vi "SelectStageTrajectory2.vi"(6 "Stage Position Limit":i32=360, 9 "Stage Speed":dbl=45.0 format="%#_13g", 10 "New Stage Position":i32, 11 "Stage Position":dbl) -> ()   [LabVIEW 2013]
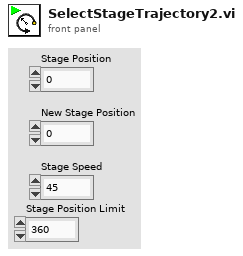
[diagram p1: front panel]
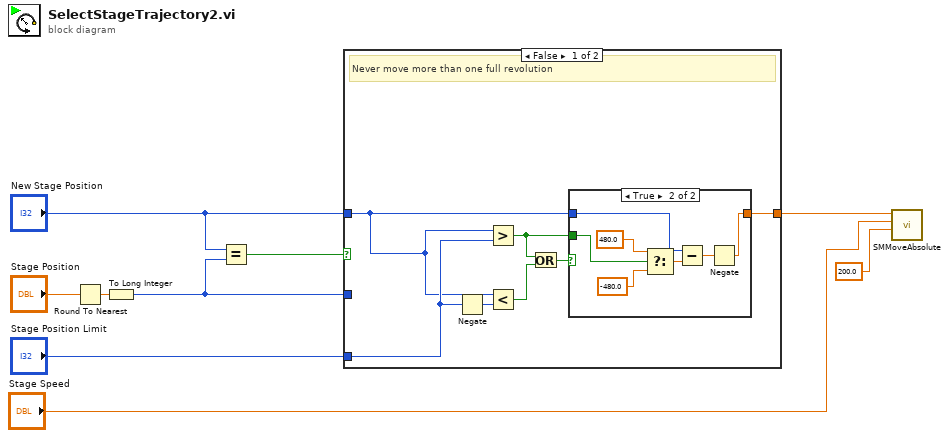
[diagram p0: block diagram]
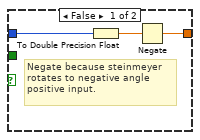
[diagram p2: hidden frame]
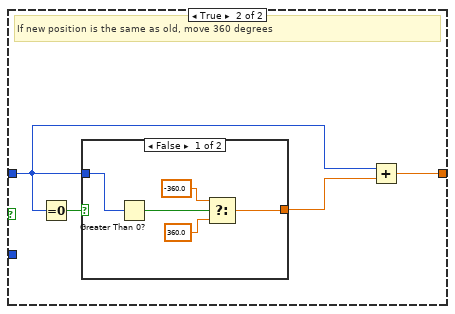
[diagram p3: hidden frame]
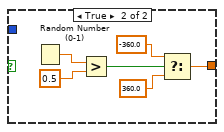
[diagram p4: hidden frame]
diagram:
  n1 = Round To Nearest(number="Stage Position") -> (nearest integer value=w7:dbl)
  n2 = To Long Integer(number=w7) -> (32bit integer=w4:i32)
  n3 = Equal?(x="New Stage Position", y=w4) -> (x = y?=w6:bool)
  n4 = case shown="False" w6 {
    tunnel: "New Stage Position" -> [w10 w28]
    tunnel: [w13 w27] -> w3
    tunnel: w4 -> [_ _]
    tunnel: "Stage Position Limit" -> [w12 _]
    frame False {
      # "Never move more than one full revolution"
      n5 = Negate(x=w12) -> (-x=w11:i32)
      n6 = Greater?(x=w10, y=w12) -> (0:w14:bool)
      n7 = Less?(x=w10, y=w11) -> (x < y?=w15:bool)
      n8 = Or(x=w14, y=w15) -> (x .or. y?=w16:bool)
      n9 = case shown="True" w16 {
        tunnel: w14 -> [_ w24]
        tunnel: w10 -> [w19 w23]
        tunnel: [w17 w20] -> w13
        frame False {
          # "Negate because steinmeyer \nrotates to negative angle \npositive input."
          n10 = To Double Precision Float(number=w19) -> (double precision float=w18:dbl)
          n11 = Negate(x=w18) -> (-x=w17:dbl)
        }
        frame True {
          n12 = Select(t=480.0, s=w24, f=-480.0) -> (s? t:f=w22:dbl)
          n13 = Subtract(x=w23, y=w22) -> (x-y=w21:dbl)
          n14 = Negate(x=w21) -> (-x=w20:dbl)
        }
      }
    }
    frame True {
      # "If new position is the same as old, move 360 degrees"
      n15 = Equal To 0?(x=w28) -> (x = 0?=w30:bool)
      n16 = case shown="False" w30 {
        tunnel: w28 -> [w35 _]
        tunnel: [w31 w36] -> w29
        frame False {
          n17 = Greater Than 0?(x=w35) -> (x > 0?=w32:bool)
          n18 = Select(t=-360.0, s=w32, f=360.0) -> (s? t:f=w31:dbl)
        }
        frame True {
          n19 = Random Number (0-1)() -> (number: 0 to 1=w41:dbl)
          n20 = Greater?(x=w41, y=0.5) -> (0:w37:bool)
          n21 = Select(t=-360.0, s=w37, f=360.0) -> (s? t:f=w36:dbl)
        }
      }
      n22 = Add(x=w28, y=w29) -> (x+y=w27:dbl)
    }
  }
  n23 = call "SMMoveAbsolute.vi"("Acceleration"=200.0, "Speed"="Stage Speed", "Position"=w3) -> ()  [unwired: 9 in]
